vi "CloseHandle.vi"(2 "error in (no error)":errorcluster, 3 "OphirRef In":T1) -> (0 "error out":errorcluster, 1 "OphirRef Out":T1)   [LabVIEW 2012]
uses:
  TypeDefs/OphirRef.ctl
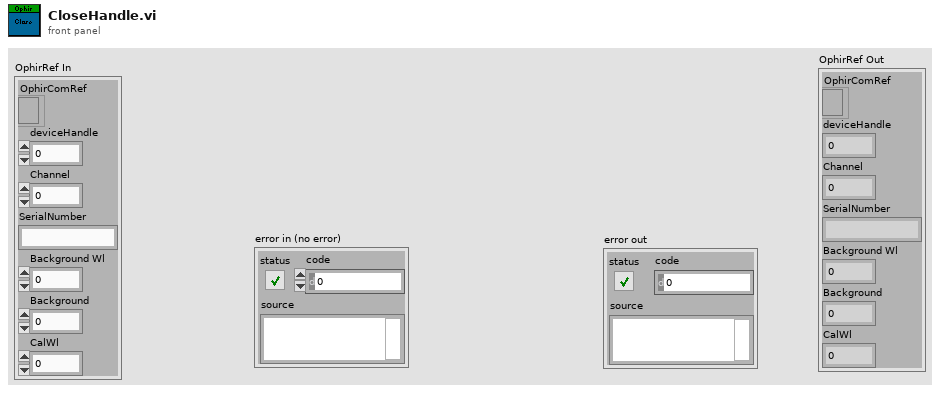
[diagram p1: front panel]
types:
  T1 = typedef "OphirRef.ctl" = cluster{"OphirComRef":refnum<k7>, "deviceHandle":i32, "Channel":i32, "SerialNumber":string, "Background Wl":dbl, "Background":dbl, "CalWl":dbl}
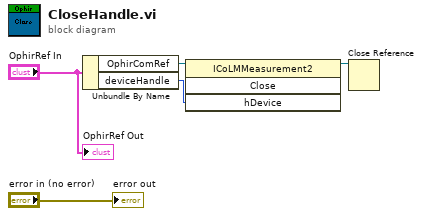
[diagram p0: block diagram]
diagram:
  n1 = Unbundle By Name("OphirRef In") -> ("OphirComRef"=w5:refnum<k7>, "deviceHandle"=w4:i32)
  n2 = invoke class="ICoLMMeasurement2" method="Close"(reference=w5, "hDevice"=w4) -> (reference out=w1:refnum<k7>)  [unwired: 2 in, 3 out]
  n3 = Close Reference(reference=w1) -> ()  [unwired: 1 in, 1 out]
  "OphirRef Out" <- "OphirRef In"
  "error out" <- "error in (no error)"
